vi "DAC timeline.vi"(1 "Plot T/F array":bool[](array[boolean]), 2 "Static DAC Array":dbl[][](array[numeric])=[[0.0, 0.0, -0.2588607594936709, 1.1708860759493671, 0.0, 0.0, 0.0, 0.0], [0.0, -0.6329113924050632, -0.2588607594936709, -0.6329113924050632, 0.0, 0.0, 0.0, 0.0], [0.0, 0.0, -0.2588607594936709, 1.1708860759493671, 0.0, 0.0, 0.0, 0.0], [0.0, 0.0, -0.2588607594936709, 0.0, 0.0, 0.0, 0.0, 0.0], [0.0, 0.0, -0.2588607594936709, 1.1708860759493671, 0.0, 0.0, 0.0, 0.0]], 3 "times":dbl[](array[numeric])) -> (0 "Timeline":T1(graph))   [LabVIEW 2017]
doc: "This vi is for plotting the Static DAC voltages as a function of time. The inputs are the Static DAC array, the 1D array of times, and a 1D array of booleans (to choose what DACs are plotted). Output is the cluster for the graph."
uses:
  globals/RIO and DAC defaults global.vi
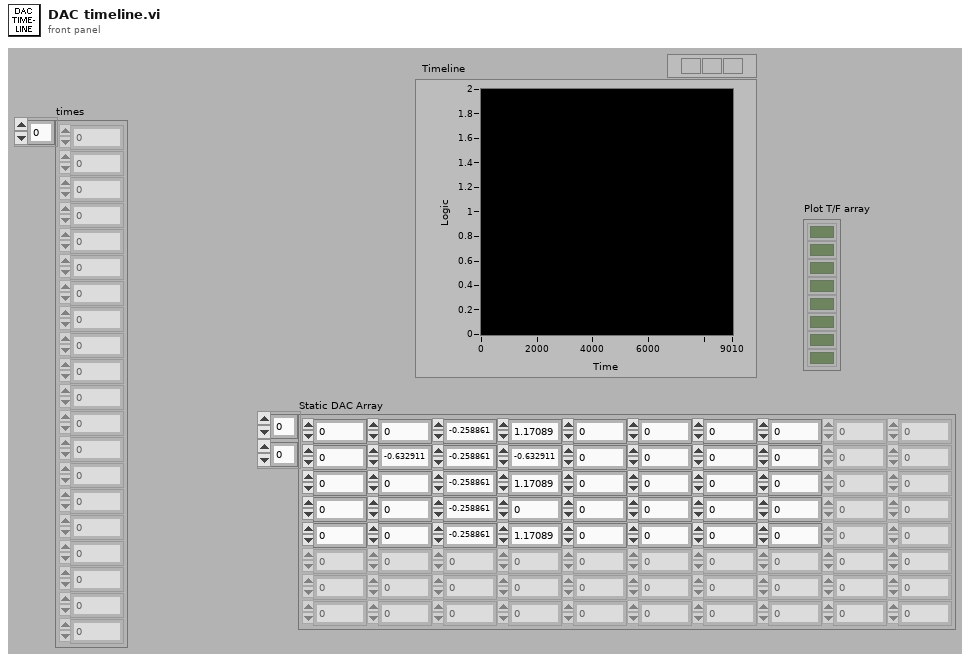
[diagram p1: front panel]
types:
  T1 = cluster{"times":dbl[], "Static DAC Array":dbl[]}[]
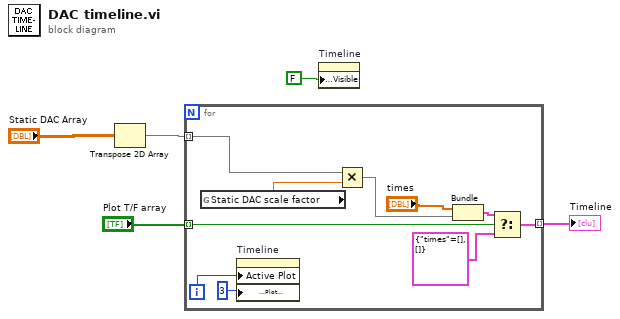
[diagram p0: block diagram]
diagram:
  n1 = Transpose 2D Array(2D array="Static DAC Array") -> (transposed array=w1:dbl[][])
  n2 = for {
    tunnel: w1 -> [w12] mode=indexing
    tunnel: [w9] -> w4 mode=indexing
    tunnel: "Plot T/F array" -> [w7] mode=indexing
    i -> [w15]
    n3 = global read "RIO and DAC defaults global.vi" "Static DAC scale factor"() -> (w6:dbl)
    n4 = property on="Timeline" class="XYGraph (strict)"("Active Plot"=w15, "Plot.Plot Interpolation"=u8 3) -> ()  [unwired: 2 in, 2 out]
    n5 = Multiply(x=w12, y=w6) -> (x*y=w11:dbl[])
    n6 = Bundle("times"="times", w11) -> (w10:cluster{"times":dbl[], dbl[]})  [unwired: 1 in]
    n7 = Select(t=w10, s=w7, f=cluster{"times":dbl[], dbl[]} {"times"=[], []} ("output cluster")) -> (s? t:f=w9:cluster{"times":dbl[], dbl[]})
  }
  "Timeline" <- w4
  n8 = property on="Timeline" class="XYGraph (strict)"("Legend:Visible"=FALSE) -> ()  [unwired: 2 in, 2 out]
